vi "Disable Scheduled Message.vi"(8 "error in (no error)":errorcluster, 11 "message handle in":u64) -> (0 "error out":errorcluster, 3 "message handle out":u64)   [LabVIEW 2020, in "Ballard ARINC 429 Hardware API.lvlib"]
doc: "Stops the transmission of a message specified by <B>message handle in</B>\n\nThe individual message may be resumed by a call to <B>Enable Scheduled Message</B>."
uses:
  Ballard ARINC 429 Hardware API.lvlib
  BTI429LV.dll
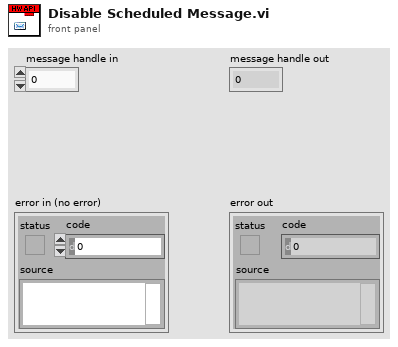
[diagram p1: front panel]
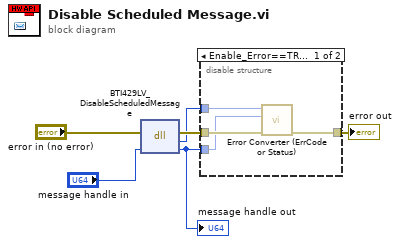
[diagram p0: block diagram]
diagram:
  n1 = dll-call lib="BTI429LV.*" fn="BTI429LV_DisableScheduledMessage"(error in="error in (no error)", "msghandle"="message handle in") -> (error out=w4:errorcluster, "return type"=w2:i32, "msghandle"=w1:u64)  [unwired: 2 in, 1 out]
  "message handle out" <- w1
  n2 = disable-structure shown="Enable_Error==TRUE" {
    disable-tunnel: w4 -> [w10 w11]
    disable-tunnel: [w9 w11] -> w3
    disable-tunnel: w2 -> [w8 _]
    disable-tunnel: w1 -> [w7 _]
    frame condition #0 {
      n3 = call "Error Converter (ErrCode or Status).vi"("error in (no error)"=w10, "handle in"=w7, "error code"=w8) -> ("error out"=w9:errorcluster)  [unwired: 8 in]
    }
    frame condition #1 (active) {
    }
  }
  "error out" <- w3
